vi "数值至布尔数组.vi"() -> ()   [LabVIEW 2014]
panel:
  out "输出簇":T1
  in  "初始化":bool
  in  "停止":bool
  in  "临时停止":bool
  in  "步信息":u16
  in  "定位运转":bool
  out "步信息":T2
  in  "返回原点":bool
  in  "控制器输入":T1
  out "人工输出":T3
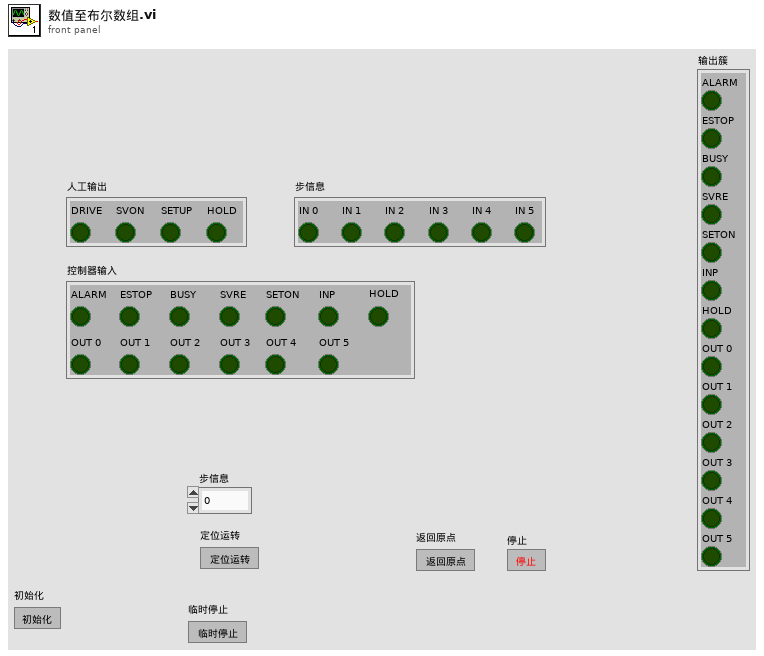
[diagram p1: front panel]
types:
  T1 = cluster{"ALARM":bool, "ESTOP":bool, "BUSY":bool, "SVRE":bool, "SETON":bool, "INP":bool, "HOLD":bool, "OUT 0":bool, "OUT 1":bool, "OUT 2":bool, "OUT 3":bool, "OUT 4":bool, "OUT 5":bool}
  T2 = cluster{"IN 0":bool, "IN 1":bool, "IN 2":bool, "IN 3":bool, "IN 4":bool, "IN 5":bool}
  T3 = cluster{"DRIVE":bool, "SVON":bool, "SETUP":bool, "HOLD":bool}
  T4 = cluster{"Boolean array[0]":bool, "Boolean array[1]":bool, "Boolean array[2]":bool, "Boolean array[3]":bool, "Boolean array[4]":bool, "Boolean array[5]":bool}
  T5 = cluster{"Boolean array[0]":bool, "Boolean array[1]":bool, "Boolean array[2]":bool, "Boolean array[3]":bool, "Boolean array[4]":bool, "Boolean array[5]":bool, "Boolean array[6]":bool, "Boolean array[7]":bool, "Boolean array[8]":bool, "Boolean array[9]":bool, "Boolean array[10]":bool, "Boolean array[11]":bool, "Boolean array[12]":bool}
  T6 = cluster{"Boolean array[0]":bool, "Boolean array[1]":bool, "Boolean array[2]":bool, "Boolean array[3]":bool}
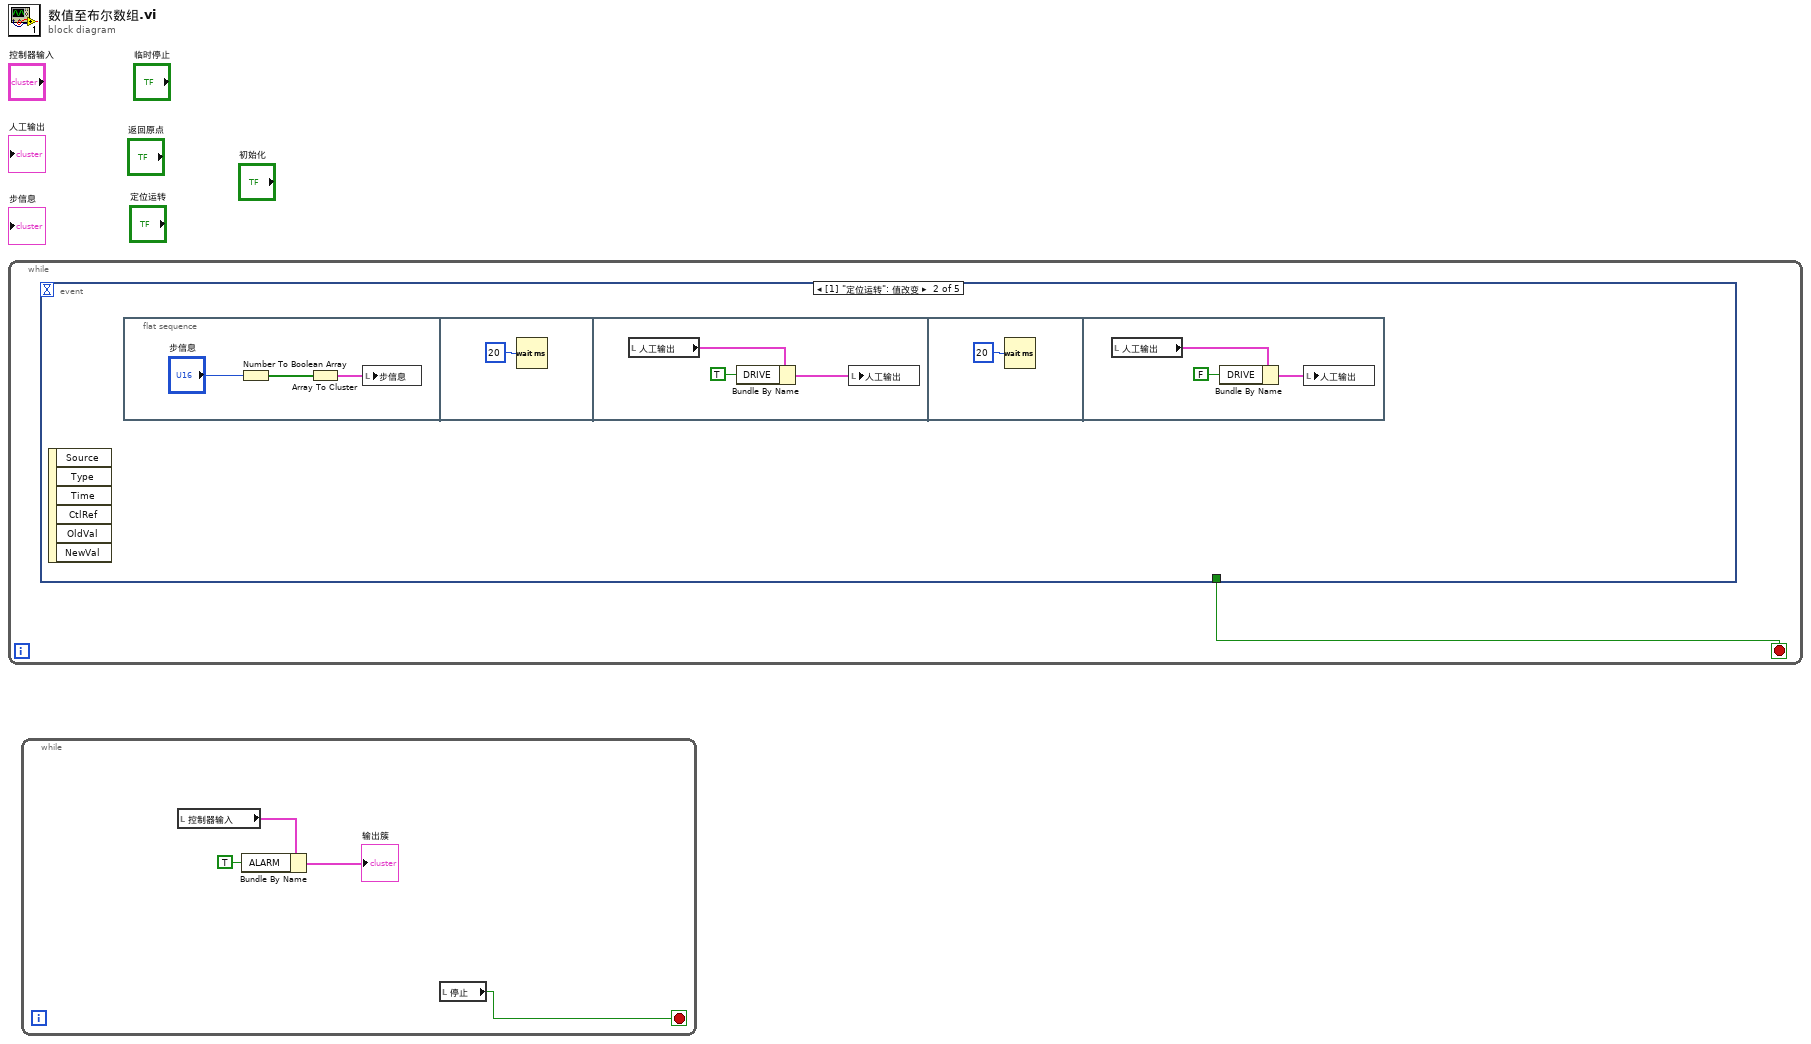
[diagram p0: block diagram]
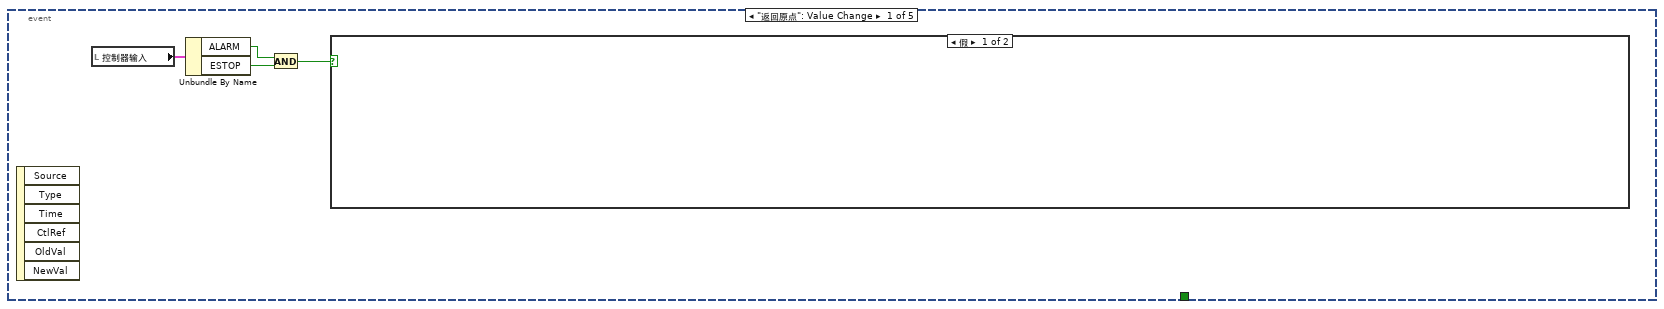
[diagram p2: hidden frame]
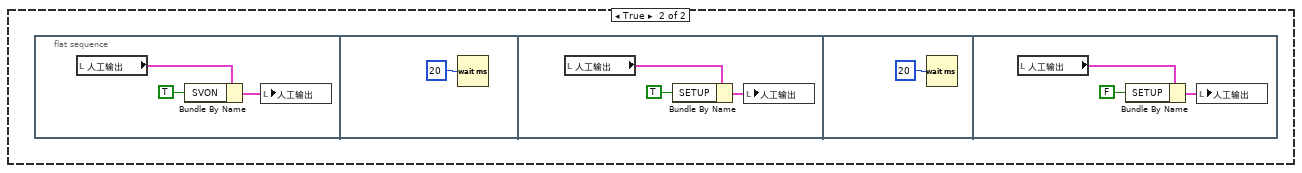
[diagram p3: hidden frame]
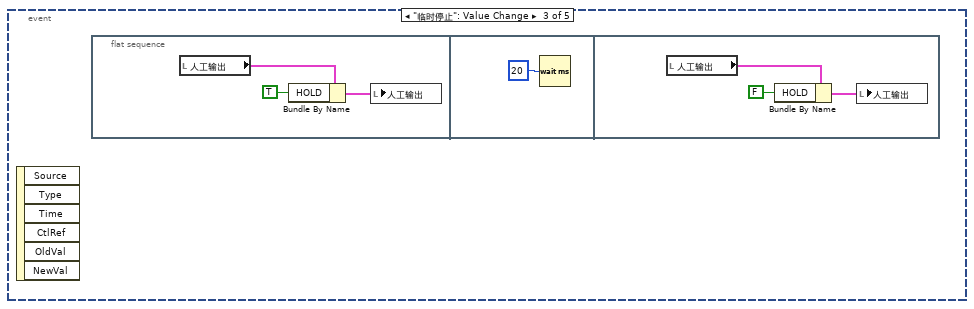
[diagram p4: hidden frame]
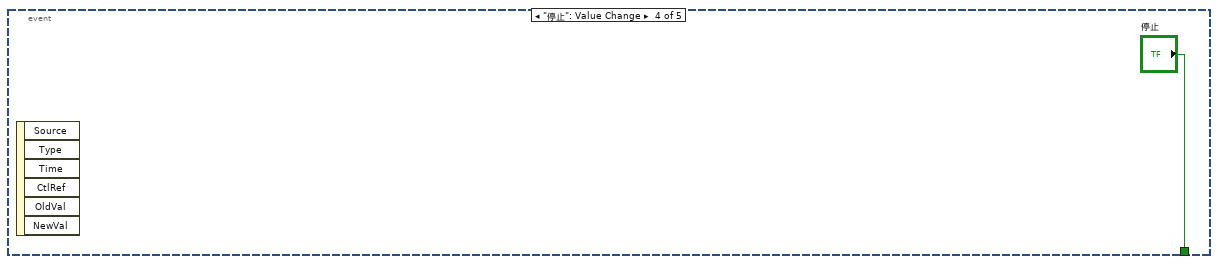
[diagram p5: hidden frame]
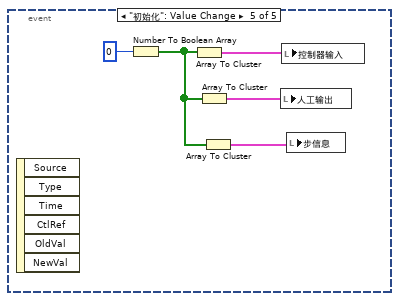
[diagram p6: hidden frame]
diagram:
  n1 = while {
    stop <- w1 stop-if-true
    n2 = event shown="[1] \"定位运转\": 值改变" {
      selector: _ -> [_ _ _ _ _]
      dyn-events: _ -> [_ _ _ _ _]
      timeout: _ -> [_ _ _ _ _]
      tunnel: [_ _ _ "停止" _] -> w1
      event "返回原点": Value Change {
        n3 = event-data() -> ()  [unwired: 1 in, 6 out]
        n4 = local read "控制器输入"() -> (w5:T1)
        n5 = Unbundle By Name(w5) -> ("ALARM"=w4:bool, "ESTOP"=w3:bool)
        n6 = And(x=w4, y=w3) -> (x .and. y?=w2:bool)
        n7 = case shown="假" w2 {
          frame False {
          }
          frame True {
            n8 = flat-sequence {
              frame #0 {
                n9 = local read "人工输出"() -> (w7:T3)
                n10 = Bundle By Name(cluster=w7, "SVON"=TRUE) -> (w8:T3)
                n11 = local write "人工输出"(w8) -> ()
              }
              frame #1 {
                n12 = Wait (ms)(milliseconds to wait=u32 20 ("等待时间（毫秒）")) -> ()  [unwired: 1 out]
              }
              frame #2 {
                n13 = local read "人工输出"() -> (w12:T3)
                n14 = Bundle By Name(cluster=w12, "SETUP"=TRUE) -> (w10:T3)
                n15 = local write "人工输出"(w10) -> ()
              }
              frame #3 {
                n16 = Wait (ms)(milliseconds to wait=u32 20 ("等待时间（毫秒）")) -> ()  [unwired: 1 out]
              }
              frame #4 {
                n17 = local read "人工输出"() -> (w16:T3)
                n18 = Bundle By Name(cluster=w16, "SETUP"=FALSE) -> (w14:T3)
                n19 = local write "人工输出"(w14) -> ()
              }
            }
          }
        }
      }
      event "定位运转": Value Change {
        n20 = event-data() -> ()  [unwired: 1 in, 6 out]
        n21 = flat-sequence {
          frame #0 {
            n22 = Number To Boolean Array(number="步信息") -> (Boolean array=w18:bool[])
            n23 = Array To Cluster(array=w18) -> (cluster=w17:T4)
            n24 = local write "步信息"(w17) -> ()
          }
          frame #1 {
            n25 = Wait (ms)(milliseconds to wait=u32 20 ("等待时间（毫秒）")) -> ()  [unwired: 1 out]
          }
          frame #2 {
            n26 = local read "人工输出"() -> (w23:T3)
            n27 = Bundle By Name(cluster=w23, "DRIVE"=TRUE) -> (w21:T3)
            n28 = local write "人工输出"(w21) -> ()
          }
          frame #3 {
            n29 = Wait (ms)(milliseconds to wait=u32 20 ("等待时间（毫秒）")) -> ()  [unwired: 1 out]
          }
          frame #4 {
            n30 = local read "人工输出"() -> (w27:T3)
            n31 = Bundle By Name(cluster=w27, "DRIVE"=FALSE) -> (w25:T3)
            n32 = local write "人工输出"(w25) -> ()
          }
        }
      }
      event "临时停止": Value Change {
        n33 = event-data() -> ()  [unwired: 1 in, 6 out]
        n34 = flat-sequence {
          frame #0 {
            n35 = local read "人工输出"() -> (w30:T3)
            n36 = Bundle By Name(cluster=w30, "HOLD"=TRUE) -> (w28:T3)
            n37 = local write "人工输出"(w28) -> ()
          }
          frame #1 {
            n38 = Wait (ms)(milliseconds to wait=u32 20 ("等待时间（毫秒）")) -> ()  [unwired: 1 out]
          }
          frame #2 {
            n39 = local read "人工输出"() -> (w34:T3)
            n40 = Bundle By Name(cluster=w34, "HOLD"=FALSE) -> (w32:T3)
            n41 = local write "人工输出"(w32) -> ()
          }
        }
      }
      event "停止": Value Change {
        n42 = event-data() -> ()  [unwired: 1 in, 6 out]
      }
      event "初始化": Value Change {
        n43 = event-data() -> ()  [unwired: 1 in, 6 out]
        n44 = Number To Boolean Array(number=u32 0 ("数字")) -> (Boolean array=w37:bool[])
        n45 = Array To Cluster(array=w37) -> (cluster=w40:T5)
        n46 = Array To Cluster(array=w37) -> (cluster=w38:T6)
        n47 = Array To Cluster(array=w37) -> (cluster=w36:T4)
        n48 = local write "人工输出"(w38) -> ()
        n49 = local write "控制器输入"(w40) -> ()
        n50 = local write "步信息"(w36) -> ()
      }
    }
  }
  n51 = while {
    stop <- w41 stop-if-true
    n52 = local read "控制器输入"() -> (w44:T1)
    n53 = Bundle By Name(cluster=w44, "ALARM"=TRUE) -> (→"输出簇":T1)
    n54 = local read "停止"() -> (w41:bool)
  }
